vi "get control.vi"(7 "error in (no error)":errorcluster, 10 "VISA In":refnum<visa-resource-name>) -> (0 "error out":errorcluster, 1 "Control?":bool, 3 "VISA out":refnum<visa-resource-name>)   [LabVIEW 2019, in "9T cmag.lvlib"]
uses:
  9T cmag.lvlib
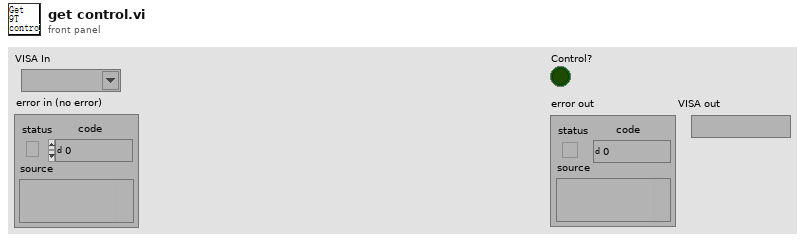
[diagram p1: front panel]
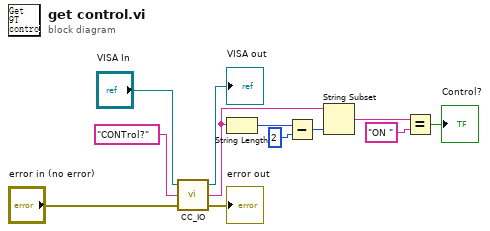
[diagram p0: block diagram]
diagram:
  n1 = call "CC_IO.vi"("error in (no error)"="error in (no error)", "Output Command"="CONTrol?" ("string"), "VISA In"="VISA In") -> ("error out"=→"error out":errorcluster, "Input String"=w5:string, "VISA out"=→"VISA out":refnum<visa-resource-name>)
  n2 = String Length(string=w5) -> (length=w4:i32)
  n3 = Subtract(x=w4, y=2) -> (x-y=w2:i32)
  n4 = String Subset(string=w5, length (rest)=w2) -> (substring=w1:string)  [unwired: 1 in]
  n5 = Equal?(x=w1, y="ON ") -> (x = y?=→"Control?":bool)
